vi "user process.vi"(8 "error in":errorcluster, 11 "Parameters to process":T2) -> (0 "error out":errorcluster, 3 "Results from processing":T1)   [LabVIEW 2017, in "Conversion runtime.lvclass"]
uses:
  Conversion runtime.lvclass
  parameter user data.ctl
  result user data.ctl
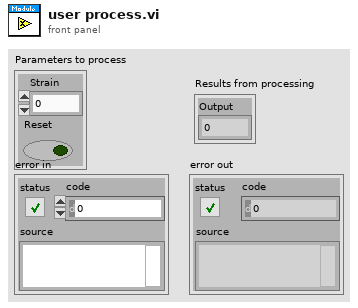
[diagram p1: front panel]
types:
  T1 = typedef "Conversion runtime.lvclass/result user data.ctl" = cluster{"Output":sgl}
  T2 = typedef "Conversion runtime.lvclass/parameter user data.ctl" = cluster{"Strain":sgl, "Reset":bool}
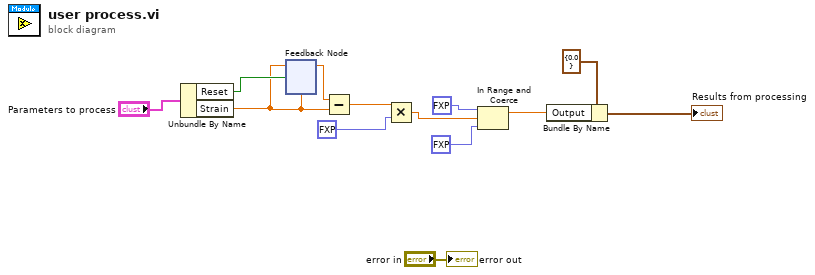
[diagram p0: block diagram]
diagram:
  n1 = Unbundle By Name("Parameters to process") -> ("Reset"=w5:bool, "Strain"=w1:sgl)
  n2 = feedback-in #1(w1, w5) -> ()
  n3 = feedback #1(w1) -> (w6:sgl)
  n4 = Subtract(x=w6, y=w1) -> (x-y=w12:sgl)
  n5 = Multiply(x=w12, y=fxp<+,32,14> 15.0) -> (x*y=w10:sgl)
  n6 = In Range and Coerce(upper limit=fxp<+/-,64,29> 10.0, x=w10, lower limit=fxp<+/-,64,29> 0.0) -> (coerced(x)=w3:sgl)  [unwired: 1 out]
  n7 = Bundle By Name(cluster=T1 {"Output"=0.0} ("Results from processing"), "Output"=w3) -> (→"Results from processing":T1)
  "error out" <- "error in"
